vi "Beamline safety test.vi"() -> ()   [LabVIEW 2013]
panel:
  out "Index Array":i32[](array[numeric])
  out "Array 2":refnum<k21>[](array[refnum])
  out "Array":refnum<k21>[](array[refnum])
  in  "stop":bool
  in  "GV 24":bool=TRUE
  in  "GV 23":bool=TRUE
  in  "GV 22":bool=TRUE
  in  "GV 21":bool=TRUE
  in  "GV 20":bool=TRUE
  in  "GV 19":bool=TRUE
  in  "GV 18":bool=TRUE
  in  "GV 17":bool=TRUE
  in  "GV 16":bool=TRUE
  in  "GV 15":bool=TRUE
  in  "GV 14":bool=TRUE
  in  "GV 13":bool=TRUE
  in  "GV 12":bool=TRUE
  in  "GV 11":bool=TRUE
  in  "GV 9":bool=TRUE
  in  "GV 10":bool=TRUE
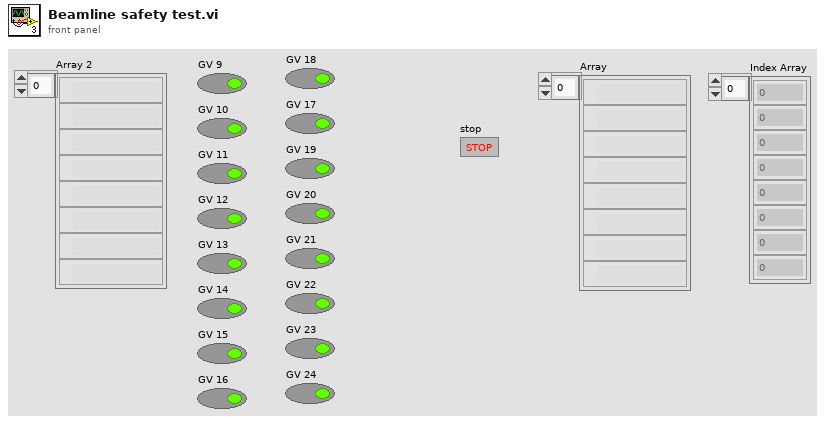
[diagram p1: front panel]
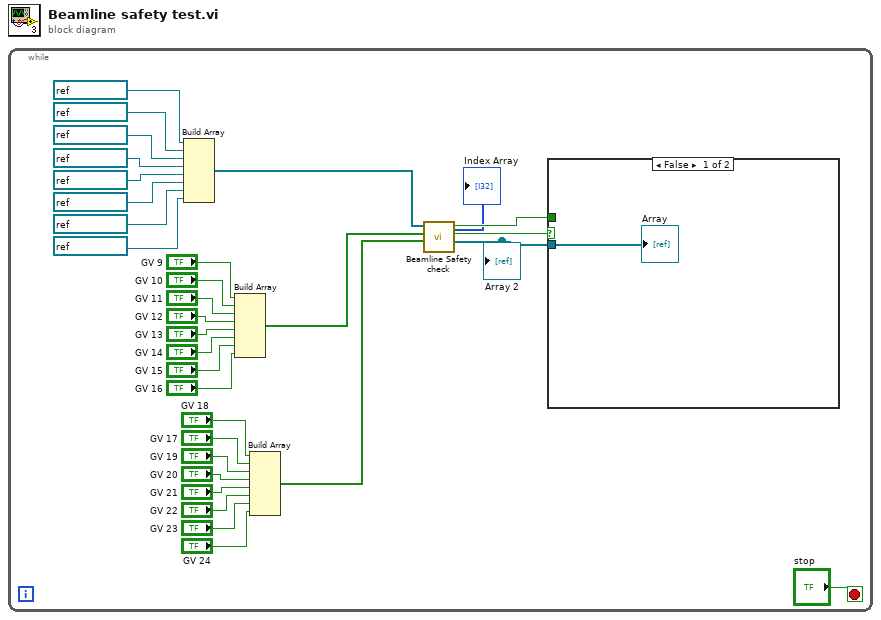
[diagram p0: block diagram]
diagram:
  n1 = while {
    stop <- "stop" stop-if-true
    n2 = Build Array(refnum<k21> "P0L0 out" ("task/channels in"), refnum<k21> "P0L1 out" ("task/channels in"), refnum<k21> "P0L2 out" ("task/channels in"), refnum<k21> "P0L3 out" ("task/channels in"), refnum<k21> "P0L4 out" ("task/channels in"), refnum<k21> "P0L5 out" ("task/channels in"), refnum<k21> "P0L6 out" ("task/channels in"), refnum<k21> "P0L7 out" ("element")) -> (w24:refnum<k21>[])
    n3 = Build Array("GV 9", "GV 10", "GV 11", "GV 12", "GV 13", "GV 14", "GV 15", "GV 16") -> (w3:bool[])
    n4 = Build Array("GV 18", "GV 17", "GV 19", "GV 20", "GV 21", "GV 22", "GV 23", "GV 24") -> (w4:bool[])
    n5 = call "Beamline Safety check.vi"("Current State Array"=w4, "Is Safe Array"=w3, "Task Array"=w24) -> ("Task Array"=w21:refnum<k21>[], "Safe conditions"=w23:bool, "Multiple Unsafe"=w22:bool, "Index Array"=→"Index Array":i32[])  [unwired: 4 in, 1 out]
    "Array 2" <- w21
    n6 = case shown="False" w23 {
      tunnel: w22 -> [_ _]
      tunnel: w21 -> [w33 _]
      frame False {
        "Array" <- w33
      }
      frame True {
      }
    }
  }
